vi "simulated CCD.vi"(8 "error in (no error)":errorcluster) -> (0 "error out":errorcluster)   [LabVIEW 2018]
uses:
  <vilib>/Utility/miscctls.llb/LVDateTimeRec.ctl
  Sim_CCD/Sim_CCD.lvclass
  Sim_CCD/Sim_CCD.lvclass/Sim_CCD.ctl
  <vilib>/addons/_JKI Toolkits/Caraya/classes/Assert/Assert Equal Value_Variant.vi
  <vilib>/addons/_JKI Toolkits/Caraya/classes/Assert/Assert Not Error.vi
  <vilib>/addons/_JKI Toolkits/Caraya/classes/Assert/Assert Almost Equal_Float.vi
  <vilib>/addons/_JKI Toolkits/Caraya/classes/Test/Test.lvclass
  <vilib>/addons/_JKI Toolkits/Caraya/classes/Assert/Assert.lvclass
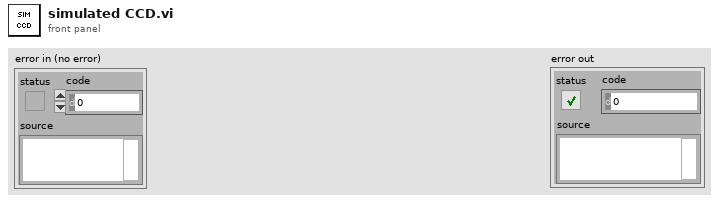
[diagram p1: front panel]
types:
  T1 = cluster{"EXPTIME":dbl, "#FRAMES":u32, "COOLER_POWER_STATUS":u16, "TEMP":i32}
  T2 = cluster{"FRAMES_DONE":u16, "CCD_STATUS":string, "CURRENT_TEMPERATURE":i16, "TEMPERATURE_STATUS":string, "FRAME_EXPOSURE_TIME":sgl, "SERIAL_NUMBER":u16, "ACQUIRING":bool, "POWER":bool, "ACS MODE":bool}
  T3 = cluster{"EXPTIME":errorcluster, "#FRAMES":errorcluster, "COOLER_POWER_STATUS":errorcluster, "TEMP":errorcluster}
  T4 = typedef "LVDateTimeRec.ctl" = cluster{"fractional second":dbl, "second":i32, "minute":i32, "hour":i32, "day of month":i32, "month":i32, "year":i32, "day of week":i32, "day of year":i32, "DST":i32}
  T5 = cluster{"Time Acq Started":u32, "Image delay":u64, "Last update - CCD config":timestamp, "SYSTEMTIME":T4, "Readout time":dbl, "Time acq finished":u32, "effective exptime":dbl}
  T6 = cluster{"PREAMP":u16, "READOUT_RATE":u16, "VERTICAL_SHIFT_SPEED":u16, "READ_MODE":u16, "VERTICAL_CLOCK_VOLTAGE":u16, "ACQUISITION_MODE":u16, "AD_CHANNEL":u16, "SHUTTER_TTL":u16, "SHUTTER_OPENING_TIME":u16, "SHUTTER_CLOSING_TIME":u16, "SHUTTER_MODE":u16, "TRIGGER_MODE":u16, "VBIN":u16, "INITIAL_LINE":u16, "INITIAL_COLUMN":u16, "FINAL_LINE":u16, "FINAL_COLUMN":u16, "HBIN":u16}
  T7 = cluster{"FRAMES_DONE":u16, "CCD_STATUS":string, "CURRENT_TEMPERATURE":i16, "TEMPERATURE_STATUS":string, "FRAME_EXPOSURE_TIME":dbl, "SERIAL_NUMBER":u16, "ACQUIRING":bool, "POWER":bool, "ACS MODE":bool}
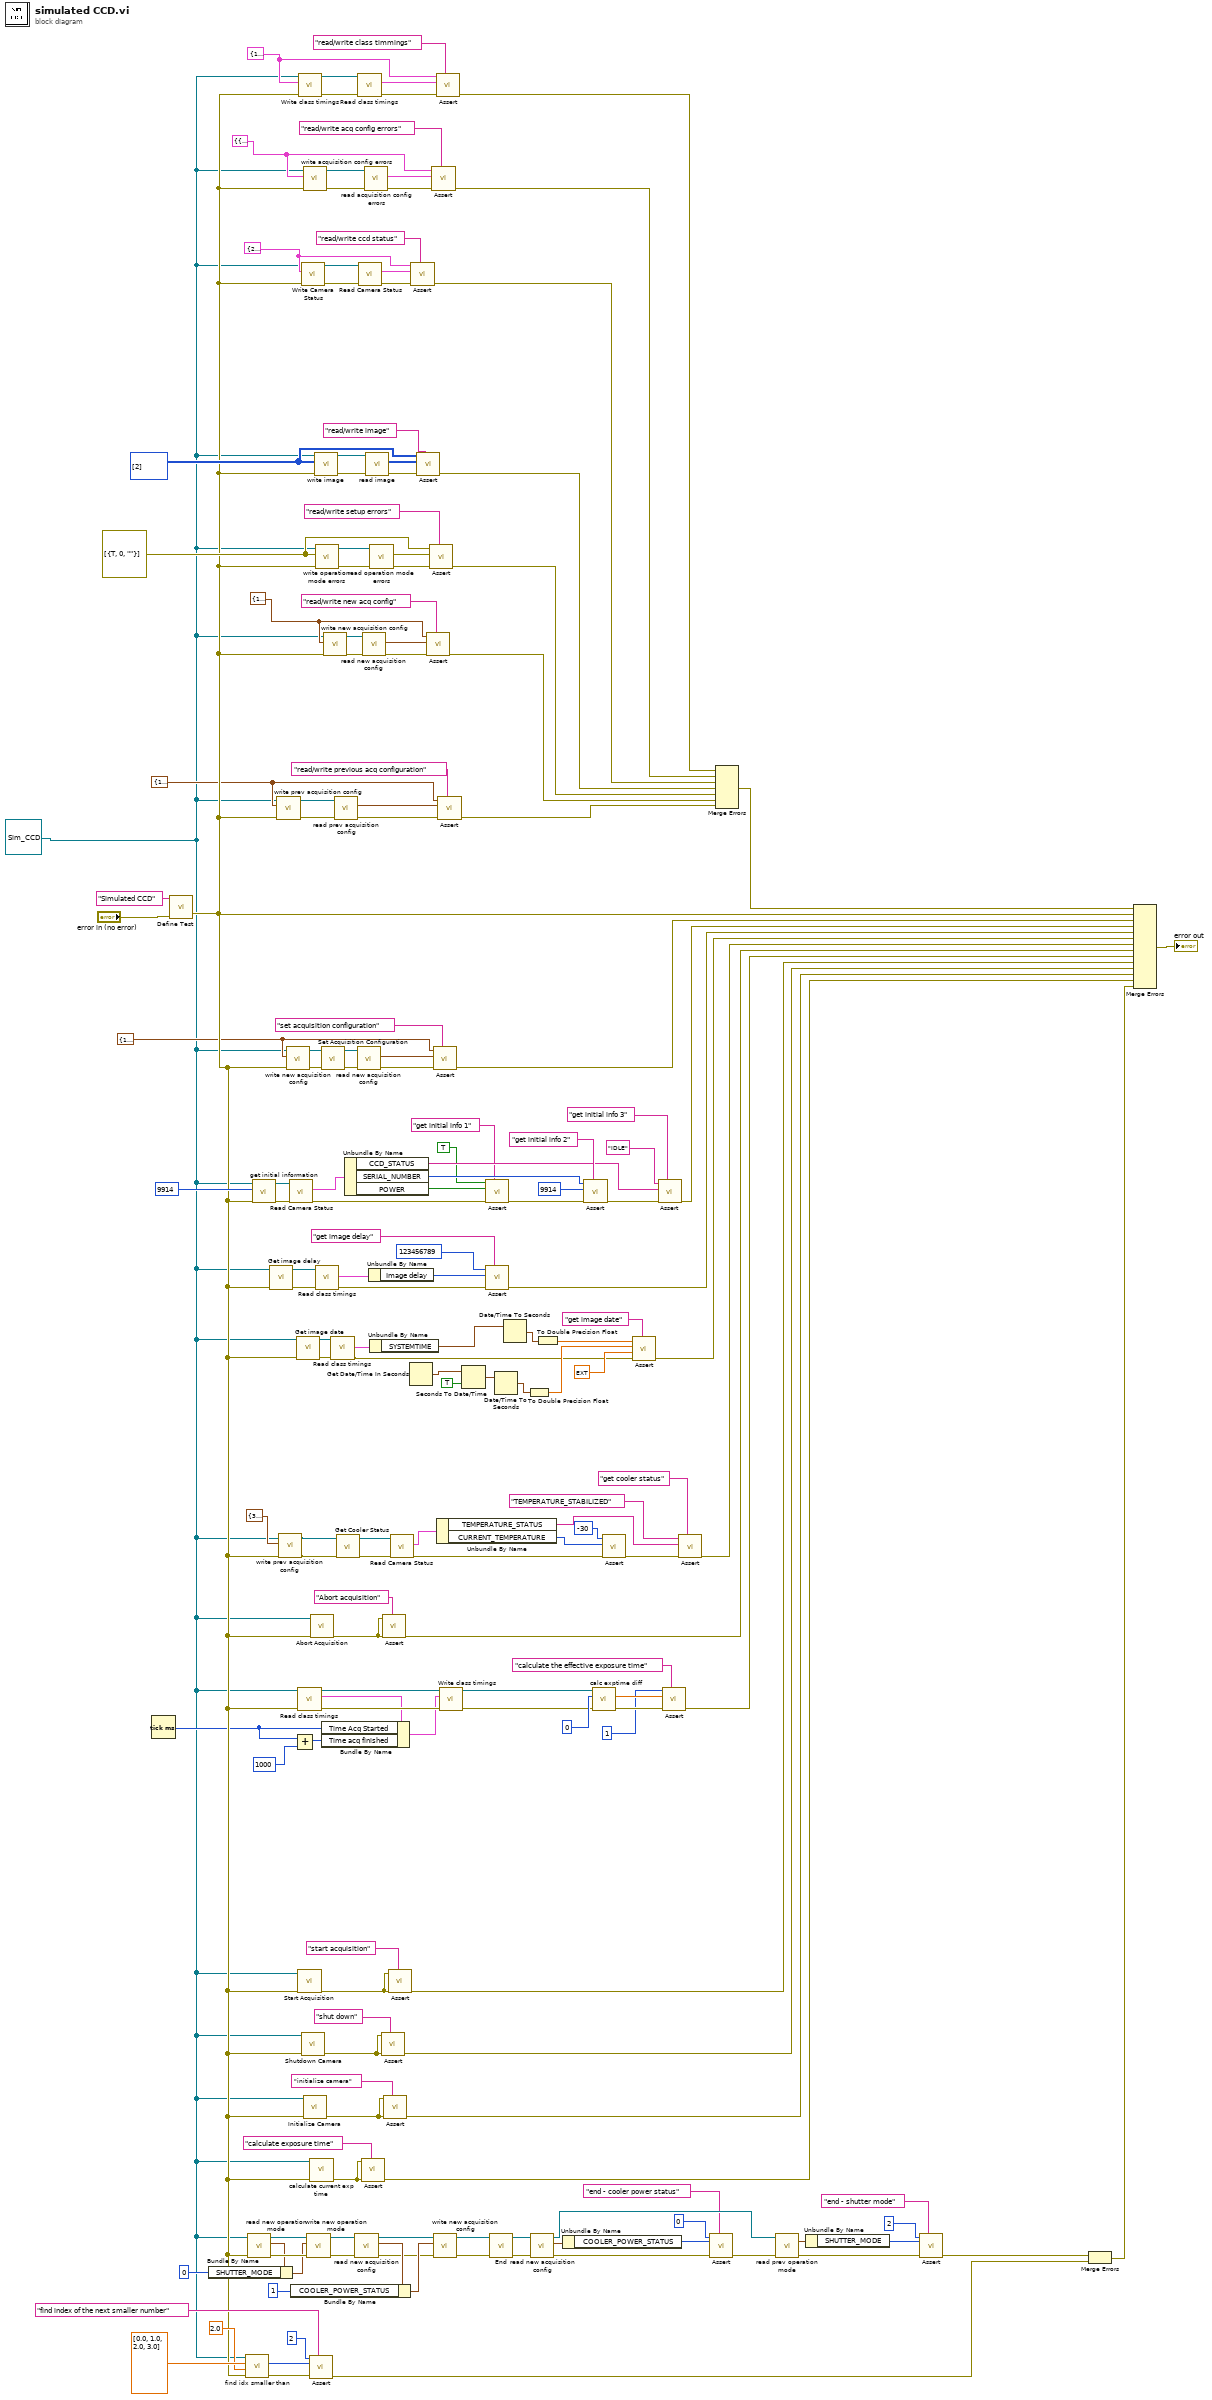
[diagram p0: block diagram]
diagram:
  w1 = refnum<class "Sim_CCD.lvclass"> refnum ("Sim_CCD.lvclass")
  w54 = T2 {"FRAMES_DONE"=2, "CCD_STATUS"="ASD", "CURRENT_TEMPERATURE"=12, "TEMPERATURE_STATUS"="ABC", "FRAME_EXPOSURE_TIME"=2.0, "SERIAL_NUMBER"=1, "ACQUIRING"=TRUE, "POWER"=TRUE, "ACS MODE"=TRUE} ("camera status")
  w12 = T3 {"EXPTIME"={"status"=TRUE, "code"=4, "source"=""}, "#FRAMES"={"status"=TRUE, "code"=3, "source"=""}, "COOLER_POWER_STATUS"={"status"=TRUE, "code"=2, "source"=""}, "TEMP"={"status"=TRUE, "code"=1, "source"=""}} ("acquisition config errors")
  w13 = T1 {"EXPTIME"=1.0, "#FRAMES"=2, "COOLER_POWER_STATUS"=1, "TEMP"=23} ("prev acquisition configuration")
  w14 = T1 {"EXPTIME"=1.0, "#FRAMES"=2, "COOLER_POWER_STATUS"=1, "TEMP"=23} ("prev acquisition configuration")
  w15 = T1 {"EXPTIME"=1.0, "#FRAMES"=2, "COOLER_POWER_STATUS"=1, "TEMP"=23} ("prev acquisition configuration")
  w59 = T5 {"Time Acq Started"=1, "Image delay"=2, "Last update - CCD config"=timestamp(0 s since 1904-01-01), "SYSTEMTIME"={"fractional second"=3.0, "second"=4, "minute"=5, "hour"=3, "day of month"=7, "month"=8, "year"=5, "day of week"=4, "day of year"=9, "DST"=6}, "Readout time"=0.0, "Time acq finished"=0, "effective exptime"=0.0} ("class timings")
  w166 = u16[][] [[2]] ("Image Graph")
  w172 = errorcluster[] [{"status"=TRUE, "code"=0, "source"=""}] ("WRITE SETUP errors")
  n1 = Tick Count (ms)() -> (millisecond timer value=w16:u32)
  n2 = call <vilib>:"Define Test.vi"("error in (no error)"="error in (no error)", "Label (VI Title)"="Simulated CCD") -> ("error out"=w24:errorcluster)  [unwired: 8 in, 1 out]
  n3 = call "find idx smaller than.vi"("error in (no error)"=w24, "Numeric"=2.0, "Array"=dbl[] [0.0, 1.0, 2.0, 3.0], "Simulated Camera in"=w1) -> ("error out"=w74:errorcluster, "index"=w73:i32)  [unwired: 5 in, 1 out]
  n4 = call "read new operation mode.vi"("error in (no error)"=w24, "CCDCamera in"=w1) -> ("error out"=w93:errorcluster, "new operation mode"=w77:T6, "CCDCamera out"=w94:refnum<class "Sim_CCD.lvclass">)  [unwired: 7 in]
  n5 = Bundle By Name(cluster=w77, "SHUTTER_MODE"=u16 0 ("COOLER_POWER_STATUS")) -> (w92:T6)
  n6 = call-dynamic "get initial information.vi"("error in (no error)"=w24, "SERN"=u16 9914 ("channel"), "Simulated_CCD_Camera in"=w1) -> ("error out"=w152:errorcluster, "Simulated_CCD_Camera out"=w151:refnum<class "Sim_CCD.lvclass">)  [unwired: 7 in]
  n7 = call-dynamic "Get image delay.vi"("error in (no error)"=w24, "Simulated_CCD_Camera in"=w1) -> ("error out"=w45:errorcluster, "Simulated_CCD_Camera out"=w44:refnum<class "Sim_CCD.lvclass">)  [unwired: 8 in]
  n8 = call "write prev acquisition config.vi"("error in (no error)"=w24, "prev acquisition configuration"=w15, "Simulated_CCD_Camera in"=w1) -> ("error out"=w48:errorcluster, "Simulated_CCD_Camera out"=w47:refnum<class "Sim_CCD.lvclass">)  [unwired: 7 in]
  n9 = call "write prev acquisition config.vi"("error in (no error)"=w24, "prev acquisition configuration"=T1 {"EXPTIME"=3.0, "#FRAMES"=4, "COOLER_POWER_STATUS"=1, "TEMP"=-30}, "Simulated_CCD_Camera in"=w1) -> ("error out"=w64:errorcluster, "Simulated_CCD_Camera out"=w65:refnum<class "Sim_CCD.lvclass">)  [unwired: 7 in]
  n10 = call "write new acquisition config.vi"("error in (no error)"=w24, "new acquisition configuration"=w14, "Simulated_CCD_Camera in"=w1) -> ("error out"=w40:errorcluster, "Simulated_CCD_Camera out"=w39:refnum<class "Sim_CCD.lvclass">)  [unwired: 7 in]
  n11 = call "Read Camera Status.vi"("error in (no error)"=w152, "CCDCamera in"=w151) -> ("error out"=w34:errorcluster, "camera status"=w150:T7)  [unwired: 7 in, 1 out]
  n12 = Add(x=w16, y=u32 1000) -> (x+y=w17:u32)
  n13 = call-dynamic "Get image date.vi"("error in (no error)"=w24, "Simulated_CCD_Camera in"=w1) -> ("error out"=w28:errorcluster, "Simulated_CCD_Camera out"=w29:refnum<class "Sim_CCD.lvclass">)  [unwired: 8 in]
  n14 = call "Read class timings.vi"("error in (no error)"=w24, "Simulated Camera in"=w1) -> ("error out"=w20:errorcluster, "class timings"=w19:T5, "Simulated Camera out"=w23:refnum<class "Sim_CCD.lvclass">)  [unwired: 7 in]
  n15 = call-dynamic "Start Acquisition.vi"("error in (no error)"=w24, "CCDCamera in"=w1) -> ("error out"=w105:errorcluster)  [unwired: 8 in, 1 out]
  n16 = call "Write class timings.vi"("error in (no error)"=w24, "class timings"=w59, "Simulated Camera in"=w1) -> ("error out"=w61:errorcluster, "Simulated Camera out"=w62:refnum<class "Sim_CCD.lvclass">)  [unwired: 7 in]
  n17 = call "Write Camera Status.vi"("error in (no error)"=w24, "camera status"=w54, "CCDCamera in"=w1) -> ("error out"=w163:errorcluster, "CCDCamera out"=w162:refnum<class "Sim_CCD.lvclass">)  [unwired: 7 in]
  n18 = call-dynamic "Shutdown Camera.vi"("error in (no error)"=w24, "CCDCamera in"=w1) -> ("error out"=w103:errorcluster)  [unwired: 8 in, 1 out]
  n19 = call "write acquisition config errors.vi"("error in (no error)"=w24, "acquisition config errors"=w12, "Simulated Camera in"=w1) -> ("error out"=w55:errorcluster, "Simulated Camera out"=w56:refnum<class "Sim_CCD.lvclass">)  [unwired: 7 in]
  n20 = call-dynamic "Initialize Camera.vi"("error in (no error)"=w24, "CCDCamera in"=w1) -> ("error out"=w101:errorcluster)  [unwired: 8 in, 1 out]
  n21 = call "write new operation mode.vi"("error in (no error)"=w93, "new operation mode"=w92, "CCDCamera in"=w94) -> ("error out"=w11:errorcluster, "CCDCamera out"=w10:refnum<class "Sim_CCD.lvclass">)  [unwired: 7 in]
  n22 = call-poly <vilib>:"Assert.vi"("Label"="find index of the next smaller number" ("format string"), "error in (no error)"=w74, "Actual"=w73, "Expected"=u16 2 ("COOLER_POWER_STATUS")) -> ("error out"=w71:errorcluster)  [unwired: 6 in, 1 out]
  n23 = call-dynamic "calculate current exp time.vi"("error in (no error)"=w24, "CCDCamera in"=w1) -> ("error out"=w66:errorcluster)  [unwired: 8 in, 1 out]
  n24 = call-dynamic "Abort Acquisition.vi"("error in (no error)"=w24, "CCDCamera in"=w1) -> ("error out"=w117:errorcluster)  [unwired: 8 in, 1 out]
  n25 = call "write image.vi"("error in (no error)"=w24, "Image Graph"=w166, "CCDCamera in"=w1) -> ("error out"=w170:errorcluster, "CCDCamera out"=w169:refnum<class "Sim_CCD.lvclass">)  [unwired: 7 in]
  n26 = call "write operation mode errors.vi"("error in (no error)"=w24, "WRITE SETUP errors"=w172, "Simulated_CCD_Camera in"=w1) -> ("error out"=w178:errorcluster, "Simulated_CCD_Camera out"=w177:refnum<class "Sim_CCD.lvclass">)  [unwired: 7 in]
  n27 = call "Read class timings.vi"("error in (no error)"=w45, "Simulated Camera in"=w44) -> ("error out"=w43:errorcluster, "class timings"=w42:T5)  [unwired: 7 in, 1 out]
  n28 = call-dynamic "Set Acquisition Configuration.vi"("error in (no error)"=w40, "CCDCamera in"=w39) -> ("error out"=w38:errorcluster, "CCDCamera out"=w37:refnum<class "Sim_CCD.lvclass">)  [unwired: 8 in]
  n29 = Bundle By Name(cluster=w19, "Time Acq Started"=w16, "Time acq finished"=w17) -> (w18:T5)
  n30 = call "write new acquisition config.vi"("error in (no error)"=w24, "new acquisition configuration"=w13, "Simulated_CCD_Camera in"=w1) -> ("error out"=w51:errorcluster, "Simulated_CCD_Camera out"=w50:refnum<class "Sim_CCD.lvclass">)  [unwired: 7 in]
  n31 = call "Read class timings.vi"("error in (no error)"=w28, "Simulated Camera in"=w29) -> ("error out"=w25:errorcluster, "class timings"=w27:T5)  [unwired: 7 in, 1 out]
  n32 = call "read prev acquisition config.vi"("error in (no error)"=w48, "Simulated_CCD_Camera in"=w47) -> ("error out"=w49:errorcluster, "prev acquisition configuration"=w46:T1)  [unwired: 7 in, 1 out]
  n33 = call-dynamic "Get Cooler Status.vi"("error in (no error)"=w64, "CCDCamera in"=w65) -> ("error out"=w127:errorcluster, "CCDCamera out"=w128:refnum<class "Sim_CCD.lvclass">)  [unwired: 8 in]
  n34 = Unbundle By Name(w150) -> ("CCD_STATUS"=w145:string, "SERIAL_NUMBER"=w149:u16, "POWER"=w32:bool)
  n35 = call "read new acquisition config.vi"("error in (no error)"=w11, "Simulated_CCD_Camera in"=w10) -> ("error out"=w5:errorcluster, "new acquisition configuration"=w7:T1, "Simulated_CCD_Camera out"=w4:refnum<class "Sim_CCD.lvclass">)  [unwired: 7 in]
  n36 = Bundle By Name(cluster=w7, "COOLER_POWER_STATUS"=u16 1) -> (w6:T1)
  n37 = call "read new acquisition config.vi"("error in (no error)"=w38, "Simulated_CCD_Camera in"=w37) -> ("error out"=w36:errorcluster, "new acquisition configuration"=w35:T1)  [unwired: 7 in, 1 out]
  n38 = call "Read class timings.vi"("error in (no error)"=w61, "Simulated Camera in"=w62) -> ("error out"=w63:errorcluster, "class timings"=w60:T5)  [unwired: 7 in, 1 out]
  n39 = call "Read Camera Status.vi"("error in (no error)"=w163, "CCDCamera in"=w162) -> ("error out"=w161:errorcluster, "camera status"=w159:T7)  [unwired: 7 in, 1 out]
  n40 = call-poly <vilib>:"Assert.vi"("Label"="calculate exposure time" ("format string"), "error in (no error)"=w66, "Not Error?"=w66) -> ("error out"=w95:errorcluster)  [unwired: 7 in, 1 out]
  n41 = call "read new acquisition config.vi"("error in (no error)"=w51, "Simulated_CCD_Camera in"=w50) -> ("error out"=w53:errorcluster, "new acquisition configuration"=w52:T1)  [unwired: 7 in, 1 out]
  n42 = call "read acquisition config errors.vi"("error in (no error)"=w55, "Simulated Camera in"=w56) -> ("error out"=w58:errorcluster, "acquisition config errors"=w57:T3)  [unwired: 7 in, 1 out]
  n43 = call "read image.vi"("error in (no error)"=w170, "CCDCamera in"=w169) -> ("error out"=w168:errorcluster, "Image Graph"=w167:u16[][])  [unwired: 7 in, 1 out]
  n44 = Unbundle By Name(w42) -> ("Image delay"=w41:u64)
  n45 = Unbundle By Name(w27) -> ("SYSTEMTIME"=w26:T4)
  n46 = call "read operation mode errors.vi"("error in (no error)"=w178, "Simulated_CCD_Camera in"=w177) -> ("error out"=w175:errorcluster, "WRITE SETUP errors"=w173:errorcluster[])  [unwired: 7 in, 1 out]
  n47 = call-poly <vilib>:"Assert.vi"("Label"="shut down" ("format string"), "error in (no error)"=w103, "Not Error?"=w103) -> ("error out"=w98:errorcluster)  [unwired: 7 in, 1 out]
  n48 = call-poly <vilib>:"Assert.vi"("Label"="Abort acquisition" ("Label (VI Title)"), "error in (no error)"=w117, "Not Error?"=w117) -> ("error out"=w115:errorcluster)  [unwired: 7 in, 1 out]
  n49 = call-poly <vilib>:"Assert.vi"("Label"="initialize camera" ("format string"), "error in (no error)"=w101, "Not Error?"=w101) -> ("error out"=w97:errorcluster)  [unwired: 7 in, 1 out]
  n50 = call-poly <vilib>:"Assert.vi"("Label"="start acquisition" ("format string"), "error in (no error)"=w105, "Not Error?"=w105) -> ("error out"=w99:errorcluster)  [unwired: 7 in, 1 out]
  n51 = call "Read Camera Status.vi"("error in (no error)"=w127, "CCDCamera in"=w128) -> ("error out"=w126:errorcluster, "camera status"=w125:T7)  [unwired: 7 in, 1 out]
  n52 = Get Date/Time In Seconds() -> (seconds since 1Jan1904=w137:timestamp)
  n53 = call-poly <vilib>:"Assert.vi"("Label"="read/write ccd status", "error in (no error)"=w161, "Actual"=w159, "Expected"=w54) -> ("error out"=w160:errorcluster)  [unwired: 6 in, 1 out]
  n54 = call-poly <vilib>:"Assert.vi"("Label"="read/write image", "error in (no error)"=w168, "Actual"=w167, "Expected"=w166) -> ("error out"=w164:errorcluster)  [unwired: 6 in, 1 out]
  n55 = call-poly <vilib>:"Assert.vi"("Label"="read/write new acq config", "error in (no error)"=w53, "Actual"=w52, "Expected"=w13) -> ("error out"=w179:errorcluster)  [unwired: 6 in, 1 out]
  n56 = call-poly <vilib>:"Assert.vi"("Label"="read/write setup errors", "error in (no error)"=w175, "Actual"=w173, "Expected"=w172) -> ("error out"=w174:errorcluster)  [unwired: 6 in, 1 out]
  n57 = call-poly <vilib>:"Assert.vi"("Label"="read/write acq config errors", "error in (no error)"=w58, "Actual"=w57, "Expected"=w12) -> ("error out"=w156:errorcluster)  [unwired: 6 in, 1 out]
  n58 = call-poly <vilib>:"Assert.vi"("Label"="set acquisition configuration" ("Label (VI Title)"), "error in (no error)"=w36, "Actual"=w35, "Expected"=w14) -> ("error out"=w155:errorcluster)  [unwired: 6 in, 1 out]
  n59 = call "write new acquisition config.vi"("error in (no error)"=w5, "new acquisition configuration"=w6, "Simulated_CCD_Camera in"=w4) -> ("error out"=w8:errorcluster, "Simulated_CCD_Camera out"=w9:refnum<class "Sim_CCD.lvclass">)  [unwired: 7 in]
  n60 = call-poly <vilib>:"Assert.vi"("Label"="read/write class timmings", "error in (no error)"=w63, "Actual"=w60, "Expected"=w59) -> ("error out"=w111:errorcluster)  [unwired: 6 in, 1 out]
  n61 = Unbundle By Name(w125) -> ("TEMPERATURE_STATUS"=w121:string, "CURRENT_TEMPERATURE"=w124:i16)
  n62 = call-poly <vilib>:"Assert.vi"("Label"="read/write previous acq configuration", "error in (no error)"=w49, "Actual"=w46, "Expected"=w15) -> ("error out"=w180:errorcluster)  [unwired: 6 in, 1 out]
  n63 = call "Write class timings.vi"("error in (no error)"=w20, "class timings"=w18, "Simulated Camera in"=w23) -> ("error out"=w21:errorcluster, "Simulated Camera out"=w22:refnum<class "Sim_CCD.lvclass">)  [unwired: 7 in]
  n64 = Seconds To Date/Time(time stamp (now)=w137, to UTC (F)=TRUE) -> (date time rec=w136:T4)
  n65 = call-poly <vilib>:"Assert.vi"("Label"="get initial info 1" ("Label (VI Title)"), "error in (no error)"=w34, "Actual"=w32, "Expected"=TRUE) -> ("error out"=w33:errorcluster)  [unwired: 6 in, 1 out]
  n66 = call-poly <vilib>:"Assert.vi"("Label"="get image delay" ("Label (VI Title)"), "error in (no error)"=w43, "Actual"=w41, "Expected"=u32 123456789 ("channel")) -> ("error out"=w139:errorcluster)  [unwired: 6 in, 1 out]
  n67 = call "End.vi"("error in (no error)"=w8, "Simulated_CCD_Camera in"=w9) -> ("error out"=w91:errorcluster, "Simulated_CCD_Camera out"=w90:refnum<class "Sim_CCD.lvclass">)  [unwired: 8 in]
  n68 = Date/Time To Seconds(2:w136) -> (0:w135:timestamp)  [unwired: 1 in]
  n69 = Date/Time To Seconds(2:w26) -> (0:w134:timestamp)  [unwired: 1 in]
  n70 = To Double Precision Float(number=w135) -> (double precision float=w132:dbl)
  n71 = call "read new acquisition config.vi"("error in (no error)"=w91, "Simulated_CCD_Camera in"=w90) -> ("error out"=w89:errorcluster, "new acquisition configuration"=w88:T1, "Simulated_CCD_Camera out"=w84:refnum<class "Sim_CCD.lvclass">)  [unwired: 7 in]
  n72 = To Double Precision Float(number=w134) -> (double precision float=w133:dbl)
  n73 = Unbundle By Name(w88) -> ("COOLER_POWER_STATUS"=w87:u16)
  n74 = call-poly <vilib>:"Assert.vi"("Label"="get initial info 2" ("Label (VI Title)"), "error in (no error)"=w33, "Actual"=u16 9914 ("channel"), "Expected"=w149) -> ("error out"=w146:errorcluster)  [unwired: 6 in, 1 out]
  n75 = call-dynamic "calc exptime diff.vi"("error in (no error)"=w21, "ACS mode"=0, "Simulated_CCD_Camera in"=w22) -> ("error out"=w109:errorcluster, "effective exptime"=w108:dbl)  [unwired: 6 in, 1 out]
  n76 = call-poly <vilib>:"Assert.vi"("error in (no error)"=w126, "Actual"=w124, "Expected"=-30 ("dimension size")) -> ("error out"=w122:errorcluster)  [unwired: 7 in, 1 out]
  n77 = call-poly <vilib>:"Assert.vi"("Label"="get image date" ("Label (VI Title)"), "error in (no error)"=w25, "Tolerance"=ext 0.1, "Actual"=w132, "Expected"=w133) -> ("error out"=w130:errorcluster)  [unwired: 5 in, 1 out]
  n78 = call-poly <vilib>:"Assert.vi"("Label"="get initial info 3" ("Label (VI Title)"), "error in (no error)"=w146, "Actual"=w145, "Expected"="IDLE" ("Label (VI Title)")) -> ("error out"=w142:errorcluster)  [unwired: 6 in, 1 out]
  n79 = call-poly <vilib>:"Assert.vi"("Label"="calculate the effective exposure time" ("Label (VI Title)"), "error in (no error)"=w109, "Actual"=w108, "Expected"=u32 1 ("y")) -> ("error out"=w110:errorcluster)  [unwired: 6 in, 1 out]
  n80 = call-poly <vilib>:"Assert.vi"("Label"="get cooler status" ("Label (VI Title)"), "error in (no error)"=w122, "Actual"=w121, "Expected"="TEMPERATURE_STABILIZED" ("Label (VI Title)")) -> ("error out"=w118:errorcluster)  [unwired: 6 in, 1 out]
  n81 = call-poly <vilib>:"Assert.vi"("Label"="end - cooler power status" ("format string"), "error in (no error)"=w89, "Actual"=w87, "Expected"=u16 0 ("SHUTTER_MODE")) -> ("error out"=w85:errorcluster)  [unwired: 6 in, 1 out]
  n82 = Merge Errors(w111, w156, w160, w164, w174, w179, w180) -> (w182:errorcluster)
  n83 = call "read prev operation mode.vi"("error in (no error)"=w85, "Simulated_CCD_Camera in"=w84) -> ("error out"=w82:errorcluster, "prev operation mode"=w83:T6)  [unwired: 7 in, 1 out]
  n84 = Unbundle By Name(w83) -> ("SHUTTER_MODE"=w81:u16)
  n85 = call-poly <vilib>:"Assert.vi"("Label"="end - shutter mode" ("format string"), "error in (no error)"=w82, "Actual"=w81, "Expected"=u16 2 ("SHUTTER_MODE")) -> ("error out"=w78:errorcluster)  [unwired: 6 in, 1 out]
  n86 = Merge Errors(w78, w71) -> (w79:errorcluster)
  n87 = Merge Errors(w182, w24, w155, w142, w139, w130, w118, w115, w110, w99, w98, w97, w95, w79) -> (→"error out":errorcluster)
